vi "Read IV_data.lvclass.vi"(8 "error in (no error)":errorcluster, 11 "IV in":refnum<class "IV.lvclass">) -> (0 "error out":errorcluster, 2 "IV_data.lvclass":refnum<class "IV_data.lvclass">, 3 "IV out":refnum<class "IV.lvclass">)   [LabVIEW 2014, in "IV.lvclass"]
uses:
  IV.lvclass
  data/IV_data.lvclass
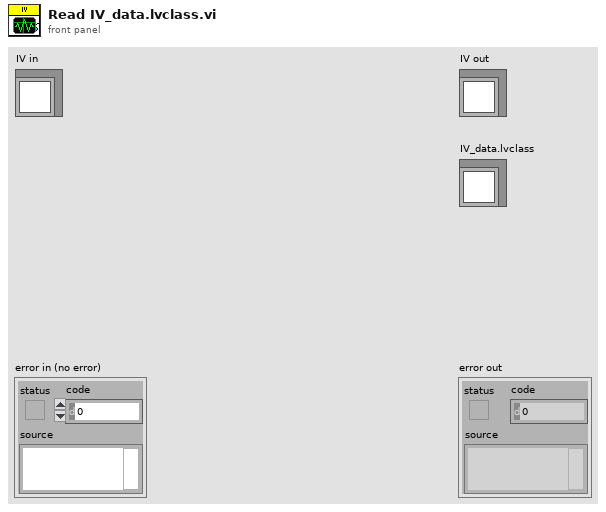
[diagram p1: front panel]
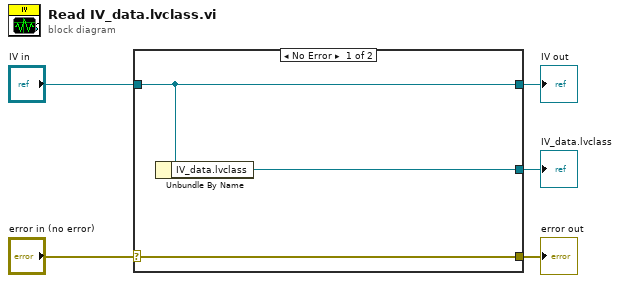
[diagram p0: block diagram]
diagram:
  n1 = case shown="No Error" "error in (no error)" {
    selector: "error in (no error)" -> [w8 w9]
    tunnel: [w8 w9] -> w4
    tunnel: [w7 w10] -> w2
    tunnel: "IV in" -> [w7 w10]
    tunnel: [w6 _] -> w1
    frame No Error {
      n2 = Unbundle By Name(w7) -> ("IV_data.lvclass"=w6:refnum<class "IV_data.lvclass">)
    }
    frame Error {
    }
  }
  "error out" <- w4
  "IV out" <- w2
  "IV_data.lvclass" <- w1
